vi "PathLength (SubVI).vi"(11 "Points":T1(array[cluster])) -> (3 "Numeric":sgl)   [LabVIEW 2014]
panel:
  out "x-1":i32
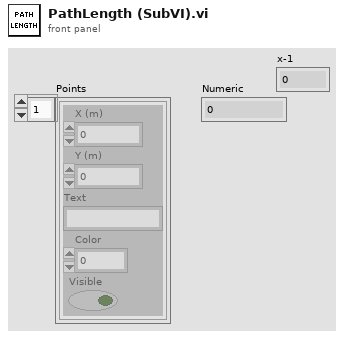
[diagram p1: front panel]
types:
  T1 = cluster{"X (m)":sgl, "Y (m)":sgl, "Text":string, "Color":u32, "Visible":bool}[]
  T2 = cluster{"X (m)":sgl, "Y (m)":sgl, "Text":string, "Color":u32, "Visible":bool}
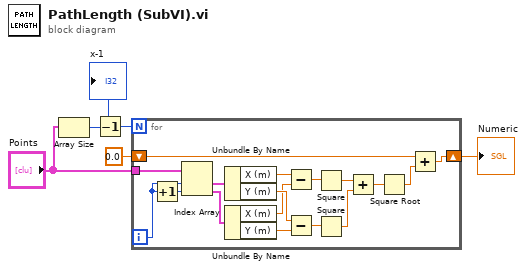
[diagram p0: block diagram]
diagram:
  n1 = Array Size(array="Points") -> (size(s)=w3:i32)
  n2 = Decrement(x=w3) -> (x-1=w2:i32)
  "x-1" <- w2
  n3 = for {
    N: w2 -> [_]
    tunnel: "Points" -> [w10]
    shift-right: [w9] -> w5
    shift-left: sgl 0.0 -> [w8]
    i -> [w7]
    n4 = Increment(x=w7) -> (x+1=w6:i32)
    n5 = Index Array(array=w10, index #1=w7, index #2=w6) -> (element #1=w22:T2, element #2=w11:T2)
    n6 = Unbundle By Name(w22) -> ("X (m)"=w12:sgl, "Y (m)"=w14:sgl)
    n7 = Unbundle By Name(w11) -> ("X (m)"=w13:sgl, "Y (m)"=w15:sgl)
    n8 = Subtract(x=w12, y=w13) -> (x-y=w17:sgl)
    n9 = Subtract(x=w14, y=w15) -> (x-y=w16:sgl)
    n10 = Square(x=w17) -> (x^2=w18:sgl)
    n11 = Square(x=w16) -> (x^2=w19:sgl)
    n12 = Add(x=w18, y=w19) -> (x+y=w20:sgl)
    n13 = Square Root(x=w20) -> (sqrt(x)=w21:sgl)
    n14 = Add(x=w8, y=w21) -> (x+y=w9:sgl)
  }
  "Numeric" <- w5
